vi "App - analyze RUS V6.vi"() -> ()   [LabVIEW 2021]
uses:
  lorentzian.ctl
  temperature sweep point.ctl
  <vilib>/Utility/miscctls.llb/LVCursorListTypeDef.ctl
  circle corners.ctl
  cursor window action.ctl
  find peak action.ctl
  follow the peak action.ctl
  slide action.ctl
  save-read action.ctl
  <vilib>/Utility/file.llb/Write To Spreadsheet File (string).vi
  complex region.ctl
  wavepacket.ctl
  cursor winow.ctl
  <vilib>/event_ctls.llb/eventvkey.ctl
  sweep file name.ctl
  single fit parameters.ctl
  omega map parameters.ctl
  plot scale state.ctl
  scale - offset gauge.ctl
  tfolder -- monotonic segment.ctl
  tfolder.ctl
  <vilib>/event_ctls.llb/lveventtype.ctl
  filter method control.ctl
  fit function selector control.ctl
  plot refs -- filter related.ctl
  peak -- parameters -- complex fit.ctl
  follow the peak control.ctl
  old slider control.ctl
  freq file read-write control.ctl
  read scan file control.ctl
panel:
  in  "magn field(T)":dbl format="%#.5f"
  in  "time (min)":dbl=1009.2833333313465
  in  "temperature(K)":dbl=69.845 format="%#.5f"
  in  "Tab : slide parameters":T1(tab)=enum."temperature folder related"
  in  "read scan file options":T2={"# columns"=3, "create bin file"=TRUE, "do not filter"=TRUE, "normalize phase"=TRUE, "read freq units"=enum."kHz"}
  in  "mapping: All":T3(ring)
  in  "slide control":T4={"in slide"=FALSE, "direction"=TRUE, "start "=FALSE, "stop"=FALSE, "next"=FALSE}
  in  "fit using":T5=enum."hyperbola"
  in  "mapping freq/gamma vs T":T3(ring)
  in  "mapping delta f vs T":T3(ring)
  in  "save/read":T6={"write to a file list"=0, "from file "="664_a", "erase"=FALSE, "load"=TRUE, "save"=TRUE, "to a file "="664_a", "read from file list"=0} {"read from file list" items=["664_a", "956_a", "1090_a"]}
  in  "follow the peak":T7={"factor"=20.0, "omega ?"=TRUE, "gamma ?"=FALSE, "max (kHz)"=30.0, "is clean"=FALSE, "acceptance"=0.5, "history - length"=10}
  in  "Tab : everything":T8(tab)
  in  "Tab : temperature folder":T9(tab)
  in  "plot when in slide":bool=TRUE
  in  "scale gauge: frequency vs T":dbl(slide)=0.9193548387096774 min=0.0 max=1.0 step=0.01 scale=0.0..1.0 scale format="%#_2g"
  out "Plot: frequency vs T":cluster{dbl[], dbl[]}[](graph)=[{array[1661 elements], array[1661 elements]}, {[14.503, 14.496, 14.494, 14.494, 14.485, 14.485, 14.487, 14.486, 14.479, 14.477, 14.476, 14.474, 14.473, 14.478, 14.475, 14.47, 14.472, 14.471, 14.469, 14.466, 14.467, 14.468, 14.463, 14.464, 14.462, 14.457, 14.457, 14.456, 14.45, 14.449, 14.446, 14.451, 14.451, 14.448, 14.449, 14.451, 14.449, 14.445, 14.447, 14.443, 14.439, 14.439, 14.439, 14.439, 14.44, 14.433, 14.434, 14.43, 14.43, 14.43, 14.434, 14.434, 14.431, 14.429, 14.426, 14.429, 14.429, 14.425, 14.426, 14.422, 14.424, 14.421, 14.418, 14.417, 14.415, 14.413, 14.414, 14.412, 14.418, 14.417, 14.412, 14.413, 14.41, 14.414, 14.408, 14.407, 14.406, 14.402, 14.4, 14.396, 14.394, 14.393, 14.39, 14.387, 14.39, 14.385, 14.384, 14.387, 14.388, 14.382, 14.384, 14.381, 14.381, 14.376, 14.375, 14.371, 14.371, 14.369, 14.369, 14.373, 14.37, 14.368, 14.366, 14.363, 14.364, 14.367, 14.363, 14.363, 14.363, 14.36, 14.361, 14.361, 14.357, 14.357, 14.355, 14.354, 14.354, 14.352, 14.349, 14.353, 14.35, 14.351, 14.351, 14.353, 14.352, 14.354, 14.354, 14.358, 14.357, 14.356, 14.356, 14.354, 14.35, 14.352, 14.354, 14.349, 14.349, 14.346], [0.0, 0.0, 0.0, 0.0, 0.0, 0.0, 0.0, 0.0, 0.0, 0.0, 0.0, 0.0, 0.0, 0.0, 0.0, 0.0, 0.0, 0.0, 0.0, 0.0, 0.0, 0.0, 0.0, 0.0, 0.0, 0.0, 0.0, 0.0, 0.0, 0.0, 0.0, 0.0, 0.0, 0.0, 0.0, 0.0, 0.0, 0.0, 0.0, 0.0, 0.0, 0.0, 0.0, 0.0, 0.0, 0.0, 0.0, 0.0, 0.0, 0.0, 0.0, 0.0, 0.0, 0.0, 0.0, 0.0, 0.0, 0.0, 0.0, 0.0, 0.0, 0.0, 0.0, 0.0, 0.0, 0.0, 0.0, 0.0, 0.0, 0.0, 0.0, 0.0, 0.0, 0.0, 0.0, 0.0, 0.0, 0.0, 0.0, 0.0, 0.0, 0.0, 0.0, 0.0, 0.0, 0.0, 0.0, 0.0, 0.0, 0.0, 0.0, 0.0, 0.0, 0.0, 0.0, 0.0, 0.0, 0.0, 0.0, 0.0, 0.0, 0.0, 0.0, 0.0, 0.0, 0.0, 0.0, 0.0, 0.0, 0.0, 0.0, 0.0, 0.0, 0.0, 0.0, 0.0, 0.0, 0.0, 0.0, 0.0, 0.0, 0.0, 0.0, 0.0, 0.0, 0.0, 0.0, 0.0, 0.0, 0.0, 0.0, 0.0, 0.0, 0.0, 0.0, 0.0, 0.0, 0.0]}, {[14.344, 14.346, 14.346, 14.348, 14.353, 14.355, 14.349, 14.351, 14.35, 14.347, 14.35, 14.349, 14.35, 14.351, 14.351, 14.352, 14.351, 14.35, 14.353, 14.354, 14.356, 14.359, 14.361, 14.36, 14.364, 14.363, 14.368, 14.367, 14.368, 14.368, 14.366, 14.369, 14.369, 14.371, 14.377, 14.377, 14.374, 14.374, 14.376, 14.375, 14.379, 14.38, 14.384, 14.382, 14.383, 14.382, 14.381, 14.386, 14.389, 14.392, 14.395, 14.397, 14.399, 14.4, 14.404, 14.405, 14.407, 14.411, 14.416, 14.42, 14.42, 14.42, 14.42, 14.426, 14.427, 14.431, 14.43, 14.431, 14.433, 14.438, 14.434, 14.438, 14.441, 14.441, 14.444, 14.44, 14.446, 14.449, 14.447, 14.448, 14.453, 14.45, 14.451, 14.449, 14.45, 14.453, 14.455, 14.456, 14.457, 14.458, 14.455, 14.459, 14.46, 14.459, 14.461, 14.465, 14.467, 14.467, 14.469, 14.467, 14.467, 14.469, 14.471, 14.473, 14.47, 14.474, 14.471, 14.471, 14.473, 14.476, 14.477, 14.479, 14.481, 14.481, 14.483, 14.483, 14.484, 14.488, 14.49, 14.491, 14.493, 14.491, 14.489, 14.491, 14.492, 14.492, 14.496, 14.498, 14.495, 14.498, 14.496, 14.503, 14.504, 14.507, 14.507, 14.508, 14.507, 14.507, 14.508, 14.509, 14.511, 14.513, 14.511, 14.512, 14.512, 14.51, 14.511, 14.511, 14.511, 14.512, 14.517, 14.515, 14.518, 14.517, 14.517, 14.518, 14.518, 14.52, 14.525, 14.521, 14.524, 14.524, 14.524, 14.523, 14.527, 14.522, 14.52, 14.522, 14.526, 14.529, 14.531, 14.534, 14.533, 14.534, 14.532, 14.536, 14.538, 14.541, 14.544, 14.545, 14.542, 14.546, 14.547, 14.544, 14.549, 14.546, 14.55, 14.556, 14.554, 14.553, 14.556, 14.556, 14.56, 14.56, 14.561, 14.562, 14.56, 14.56, 14.561, 14.563, 14.564, 14.572, 14.568, 14.565, 14.569, 14.577, 14.571, 14.58, 14.578, 14.579, 14.581, 14.58, 14.577, 14.58, 14.583, 14.582, 14.584, 14.584, 14.585, 14.585, 14.585, 14.585, 14.587, 14.593, 14.595, 14.597, 14.595, 14.597, 14.595, 14.597, 14.597, 14.599, 14.599, 14.599, 14.601, 14.605, 14.604, 14.606, 14.606, 14.609, 14.613, 14.614, 14.619, 14.618, 14.62, 14.621, 14.623, 14.624, 14.628, 14.625, 14.628, 14.63, 14.63, 14.635, 14.636, 14.637, 14.639, 14.64, 14.641, 14.644, 14.65, 14.65, 14.654, 14.654, 14.657, 14.659, 14.66, 14.661, 14.664, 14.668, 14.669, 14.673, 14.673, 14.673, 14.676, 14.678, 14.678, 14.681, 14.682, 14.685, 14.689, 14.687, 14.688, 14.693, 14.693, 14.696, 14.697, 14.697, 14.699, 14.702, 14.706, 14.708, 14.703, 14.705, 14.708, 14.709, 14.714, 14.719, 14.717, 14.723, 14.725, 14.727, 14.732, 14.737, 14.737, 14.739, 14.744, 14.747, 14.75, 14.751, 14.757, 14.754, 14.762, 14.757, 14.761, 14.768, 14.764, 14.769, 14.773, 14.772, 14.778, 14.778, 14.778, 14.784, 14.784, 14.784, 14.789, 14.788, 14.791, 14.793, 14.796, 14.797, 14.8, 14.807, 14.806, 14.808, 14.812, 14.814, 14.82, 14.816], [0.0, 0.0, 0.0, 0.0, 0.0, 0.0, 0.0, 0.0, 0.0, 0.0, 0.0, 0.0, 0.0, 0.0, 0.0, 0.0, 0.0, 0.0, 0.0, 0.0, 0.0, 0.0, 0.0, 0.0, 0.0, 0.0, 0.0, 0.0, 0.0, 0.0, 0.0, 0.0, 0.0, 0.0, 0.0, 0.0, 0.0, 0.0, 0.0, 0.0, 0.0, 0.0, 0.0, 0.0, 0.0, 0.0, 0.0, 0.0, 0.0, 0.0, 0.0, 0.0, 0.0, 0.0, 0.0, 0.0, 0.0, 0.0, 0.0, 0.0, 0.0, 0.0, 0.0, 0.0, 0.0, 0.0, 0.0, 0.0, 0.0, 0.0, 0.0, 0.0, 0.0, 0.0, 0.0, 0.0, 0.0, 0.0, 0.0, 0.0, 0.0, 0.0, 0.0, 0.0, 0.0, 0.0, 0.0, 0.0, 0.0, 0.0, 0.0, 0.0, 0.0, 0.0, 0.0, 0.0, 0.0, 0.0, 0.0, 0.0, 0.0, 0.0, 0.0, 0.0, 0.0, 0.0, 0.0, 0.0, 0.0, 0.0, 0.0, 0.0, 0.0, 0.0, 0.0, 0.0, 0.0, 0.0, 0.0, 0.0, 0.0, 0.0, 0.0, 0.0, 0.0, 0.0, 0.0, 0.0, 0.0, 0.0, 0.0, 0.0, 0.0, 0.0, 0.0, 0.0, 0.0, 0.0, 0.0, 0.0, 0.0, 0.0, 0.0, 0.0, 0.0, 0.0, 0.0, 0.0, 0.0, 0.0, 0.0, 0.0, 0.0, 0.0, 0.0, 0.0, 0.0, 0.0, 0.0, 0.0, 0.0, 0.0, 0.0, 0.0, 0.0, 0.0, 0.0, 0.0, 0.0, 0.0, 0.0, 0.0, 0.0, 0.0, 0.0, 0.0, 0.0, 0.0, 0.0, 0.0, 0.0, 0.0, 0.0, 0.0, 0.0, 0.0, 0.0, 0.0, 0.0, 0.0, 0.0, 0.0, 0.0, 0.0, 0.0, 0.0, 0.0, 0.0, 0.0, 0.0, 0.0, 0.0, 0.0, 0.0, 0.0, 0.0, 0.0, 0.0, 0.0, 0.0, 0.0, 0.0, 0.0, 0.0, 0.0, 0.0, 0.0, 0.0, 0.0, 0.0, 0.0, 0.0, 0.0, 0.0, 0.0, 0.0, 0.0, 0.0, 0.0, 0.0, 0.0, 0.0, 0.0, 0.0, 0.0, 0.0, 0.0, 0.0, 0.0, 0.0, 0.0, 0.0, 0.0, 0.0, 0.0, 0.0, 0.0, 0.0, 0.0, 0.0, 0.0, 0.0, 0.0, 0.0, 0.0, 0.0, 0.0, 0.0, 0.0, 0.0, 0.0, 0.0, 0.0, 0.0, 0.0, 0.0, 0.0, 0.0, 0.0, 0.0, 0.0, 0.0, 0.0, 0.0, 0.0, 0.0, 0.0, 0.0, 0.0, 0.0, 0.0, 0.0, 0.0, 0.0, 0.0, 0.0, 0.0, 0.0, 0.0, 0.0, 0.0, 0.0, 0.0, 0.0, 0.0, 0.0, 0.0, 0.0, 0.0, 0.0, 0.0, 0.0, 0.0, 0.0, 0.0, 0.0, 0.0, 0.0, 0.0, 0.0, 0.0, 0.0, 0.0, 0.0, 0.0, 0.0, 0.0, 0.0, 0.0, 0.0, 0.0, 0.0, 0.0, 0.0, 0.0, 0.0, 0.0, 0.0, 0.0, 0.0, 0.0, 0.0, 0.0, 0.0, 0.0, 0.0, 0.0, 0.0, 0.0, 0.0]}]
  out "Plot: attenuation vs T":cluster{dbl[], dbl[]}[](graph)=[{array[1661 elements], array[1661 elements]}, {[14.503, 14.496, 14.494, 14.494, 14.485, 14.485, 14.487, 14.486, 14.479, 14.477, 14.476, 14.474, 14.473, 14.478, 14.475, 14.47, 14.472, 14.471, 14.469, 14.466, 14.467, 14.468, 14.463, 14.464, 14.462, 14.457, 14.457, 14.456, 14.45, 14.449, 14.446, 14.451, 14.451, 14.448, 14.449, 14.451, 14.449, 14.445, 14.447, 14.443, 14.439, 14.439, 14.439, 14.439, 14.44, 14.433, 14.434, 14.43, 14.43, 14.43, 14.434, 14.434, 14.431, 14.429, 14.426, 14.429, 14.429, 14.425, 14.426, 14.422, 14.424, 14.421, 14.418, 14.417, 14.415, 14.413, 14.414, 14.412, 14.418, 14.417, 14.412, 14.413, 14.41, 14.414, 14.408, 14.407, 14.406, 14.402, 14.4, 14.396, 14.394, 14.393, 14.39, 14.387, 14.39, 14.385, 14.384, 14.387, 14.388, 14.382, 14.384, 14.381, 14.381, 14.376, 14.375, 14.371, 14.371, 14.369, 14.369, 14.373, 14.37, 14.368, 14.366, 14.363, 14.364, 14.367, 14.363, 14.363, 14.363, 14.36, 14.361, 14.361, 14.357, 14.357, 14.355, 14.354, 14.354, 14.352, 14.349, 14.353, 14.35, 14.351, 14.351, 14.353, 14.352, 14.354, 14.354, 14.358, 14.357, 14.356, 14.356, 14.354, 14.35, 14.352, 14.354, 14.349, 14.349, 14.346], [0.0, 0.0, 0.0, 0.0, 0.0, 0.0, 0.0, 0.0, 0.0, 0.0, 0.0, 0.0, 0.0, 0.0, 0.0, 0.0, 0.0, 0.0, 0.0, 0.0, 0.0, 0.0, 0.0, 0.0, 0.0, 0.0, 0.0, 0.0, 0.0, 0.0, 0.0, 0.0, 0.0, 0.0, 0.0, 0.0, 0.0, 0.0, 0.0, 0.0, 0.0, 0.0, 0.0, 0.0, 0.0, 0.0, 0.0, 0.0, 0.0, 0.0, 0.0, 0.0, 0.0, 0.0, 0.0, 0.0, 0.0, 0.0, 0.0, 0.0, 0.0, 0.0, 0.0, 0.0, 0.0, 0.0, 0.0, 0.0, 0.0, 0.0, 0.0, 0.0, 0.0, 0.0, 0.0, 0.0, 0.0, 0.0, 0.0, 0.0, 0.0, 0.0, 0.0, 0.0, 0.0, 0.0, 0.0, 0.0, 0.0, 0.0, 0.0, 0.0, 0.0, 0.0, 0.0, 0.0, 0.0, 0.0, 0.0, 0.0, 0.0, 0.0, 0.0, 0.0, 0.0, 0.0, 0.0, 0.0, 0.0, 0.0, 0.0, 0.0, 0.0, 0.0, 0.0, 0.0, 0.0, 0.0, 0.0, 0.0, 0.0, 0.0, 0.0, 0.0, 0.0, 0.0, 0.0, 0.0, 0.0, 0.0, 0.0, 0.0, 0.0, 0.0, 0.0, 0.0, 0.0, 0.0]}, {[14.344, 14.346, 14.346, 14.348, 14.353, 14.355, 14.349, 14.351, 14.35, 14.347, 14.35, 14.349, 14.35, 14.351, 14.351, 14.352, 14.351, 14.35, 14.353, 14.354, 14.356, 14.359, 14.361, 14.36, 14.364, 14.363, 14.368, 14.367, 14.368, 14.368, 14.366, 14.369, 14.369, 14.371, 14.377, 14.377, 14.374, 14.374, 14.376, 14.375, 14.379, 14.38, 14.384, 14.382, 14.383, 14.382, 14.381, 14.386, 14.389, 14.392, 14.395, 14.397, 14.399, 14.4, 14.404, 14.405, 14.407, 14.411, 14.416, 14.42, 14.42, 14.42, 14.42, 14.426, 14.427, 14.431, 14.43, 14.431, 14.433, 14.438, 14.434, 14.438, 14.441, 14.441, 14.444, 14.44, 14.446, 14.449, 14.447, 14.448, 14.453, 14.45, 14.451, 14.449, 14.45, 14.453, 14.455, 14.456, 14.457, 14.458, 14.455, 14.459, 14.46, 14.459, 14.461, 14.465, 14.467, 14.467, 14.469, 14.467, 14.467, 14.469, 14.471, 14.473, 14.47, 14.474, 14.471, 14.471, 14.473, 14.476, 14.477, 14.479, 14.481, 14.481, 14.483, 14.483, 14.484, 14.488, 14.49, 14.491, 14.493, 14.491, 14.489, 14.491, 14.492, 14.492, 14.496, 14.498, 14.495, 14.498, 14.496, 14.503, 14.504, 14.507, 14.507, 14.508, 14.507, 14.507, 14.508, 14.509, 14.511, 14.513, 14.511, 14.512, 14.512, 14.51, 14.511, 14.511, 14.511, 14.512, 14.517, 14.515, 14.518, 14.517, 14.517, 14.518, 14.518, 14.52, 14.525, 14.521, 14.524, 14.524, 14.524, 14.523, 14.527, 14.522, 14.52, 14.522, 14.526, 14.529, 14.531, 14.534, 14.533, 14.534, 14.532, 14.536, 14.538, 14.541, 14.544, 14.545, 14.542, 14.546, 14.547, 14.544, 14.549, 14.546, 14.55, 14.556, 14.554, 14.553, 14.556, 14.556, 14.56, 14.56, 14.561, 14.562, 14.56, 14.56, 14.561, 14.563, 14.564, 14.572, 14.568, 14.565, 14.569, 14.577, 14.571, 14.58, 14.578, 14.579, 14.581, 14.58, 14.577, 14.58, 14.583, 14.582, 14.584, 14.584, 14.585, 14.585, 14.585, 14.585, 14.587, 14.593, 14.595, 14.597, 14.595, 14.597, 14.595, 14.597, 14.597, 14.599, 14.599, 14.599, 14.601, 14.605, 14.604, 14.606, 14.606, 14.609, 14.613, 14.614, 14.619, 14.618, 14.62, 14.621, 14.623, 14.624, 14.628, 14.625, 14.628, 14.63, 14.63, 14.635, 14.636, 14.637, 14.639, 14.64, 14.641, 14.644, 14.65, 14.65, 14.654, 14.654, 14.657, 14.659, 14.66, 14.661, 14.664, 14.668, 14.669, 14.673, 14.673, 14.673, 14.676, 14.678, 14.678, 14.681, 14.682, 14.685, 14.689, 14.687, 14.688, 14.693, 14.693, 14.696, 14.697, 14.697, 14.699, 14.702, 14.706, 14.708, 14.703, 14.705, 14.708, 14.709, 14.714, 14.719, 14.717, 14.723, 14.725, 14.727, 14.732, 14.737, 14.737, 14.739, 14.744, 14.747, 14.75, 14.751, 14.757, 14.754, 14.762, 14.757, 14.761, 14.768, 14.764, 14.769, 14.773, 14.772, 14.778, 14.778, 14.778, 14.784, 14.784, 14.784, 14.789, 14.788, 14.791, 14.793, 14.796, 14.797, 14.8, 14.807, 14.806, 14.808, 14.812, 14.814, 14.82, 14.816], [0.0, 0.0, 0.0, 0.0, 0.0, 0.0, 0.0, 0.0, 0.0, 0.0, 0.0, 0.0, 0.0, 0.0, 0.0, 0.0, 0.0, 0.0, 0.0, 0.0, 0.0, 0.0, 0.0, 0.0, 0.0, 0.0, 0.0, 0.0, 0.0, 0.0, 0.0, 0.0, 0.0, 0.0, 0.0, 0.0, 0.0, 0.0, 0.0, 0.0, 0.0, 0.0, 0.0, 0.0, 0.0, 0.0, 0.0, 0.0, 0.0, 0.0, 0.0, 0.0, 0.0, 0.0, 0.0, 0.0, 0.0, 0.0, 0.0, 0.0, 0.0, 0.0, 0.0, 0.0, 0.0, 0.0, 0.0, 0.0, 0.0, 0.0, 0.0, 0.0, 0.0, 0.0, 0.0, 0.0, 0.0, 0.0, 0.0, 0.0, 0.0, 0.0, 0.0, 0.0, 0.0, 0.0, 0.0, 0.0, 0.0, 0.0, 0.0, 0.0, 0.0, 0.0, 0.0, 0.0, 0.0, 0.0, 0.0, 0.0, 0.0, 0.0, 0.0, 0.0, 0.0, 0.0, 0.0, 0.0, 0.0, 0.0, 0.0, 0.0, 0.0, 0.0, 0.0, 0.0, 0.0, 0.0, 0.0, 0.0, 0.0, 0.0, 0.0, 0.0, 0.0, 0.0, 0.0, 0.0, 0.0, 0.0, 0.0, 0.0, 0.0, 0.0, 0.0, 0.0, 0.0, 0.0, 0.0, 0.0, 0.0, 0.0, 0.0, 0.0, 0.0, 0.0, 0.0, 0.0, 0.0, 0.0, 0.0, 0.0, 0.0, 0.0, 0.0, 0.0, 0.0, 0.0, 0.0, 0.0, 0.0, 0.0, 0.0, 0.0, 0.0, 0.0, 0.0, 0.0, 0.0, 0.0, 0.0, 0.0, 0.0, 0.0, 0.0, 0.0, 0.0, 0.0, 0.0, 0.0, 0.0, 0.0, 0.0, 0.0, 0.0, 0.0, 0.0, 0.0, 0.0, 0.0, 0.0, 0.0, 0.0, 0.0, 0.0, 0.0, 0.0, 0.0, 0.0, 0.0, 0.0, 0.0, 0.0, 0.0, 0.0, 0.0, 0.0, 0.0, 0.0, 0.0, 0.0, 0.0, 0.0, 0.0, 0.0, 0.0, 0.0, 0.0, 0.0, 0.0, 0.0, 0.0, 0.0, 0.0, 0.0, 0.0, 0.0, 0.0, 0.0, 0.0, 0.0, 0.0, 0.0, 0.0, 0.0, 0.0, 0.0, 0.0, 0.0, 0.0, 0.0, 0.0, 0.0, 0.0, 0.0, 0.0, 0.0, 0.0, 0.0, 0.0, 0.0, 0.0, 0.0, 0.0, 0.0, 0.0, 0.0, 0.0, 0.0, 0.0, 0.0, 0.0, 0.0, 0.0, 0.0, 0.0, 0.0, 0.0, 0.0, 0.0, 0.0, 0.0, 0.0, 0.0, 0.0, 0.0, 0.0, 0.0, 0.0, 0.0, 0.0, 0.0, 0.0, 0.0, 0.0, 0.0, 0.0, 0.0, 0.0, 0.0, 0.0, 0.0, 0.0, 0.0, 0.0, 0.0, 0.0, 0.0, 0.0, 0.0, 0.0, 0.0, 0.0, 0.0, 0.0, 0.0, 0.0, 0.0, 0.0, 0.0, 0.0, 0.0, 0.0, 0.0, 0.0, 0.0, 0.0, 0.0, 0.0, 0.0, 0.0, 0.0, 0.0, 0.0, 0.0, 0.0, 0.0, 0.0, 0.0, 0.0, 0.0, 0.0, 0.0, 0.0, 0.0, 0.0, 0.0, 0.0, 0.0, 0.0]}]
  in  "Sweep folder path":path=path "D:/Data/Ultrasound/LSCO/LSCO22__130814c/5_Cooling_2nd_try"
  out "Plot: Time":cluster{dbl[], dbl[]}[](graph)
  out "Plot: delta f":cluster{dbl[], dbl[]}[](graph)=[{array[1661 elements], array[1661 elements]}, {[14.503, 14.496, 14.494, 14.494, 14.485, 14.485, 14.487, 14.486, 14.479, 14.477, 14.476, 14.474, 14.473, 14.478, 14.475, 14.47, 14.472, 14.471, 14.469, 14.466, 14.467, 14.468, 14.463, 14.464, 14.462, 14.457, 14.457, 14.456, 14.45, 14.449, 14.446, 14.451, 14.451, 14.448, 14.449, 14.451, 14.449, 14.445, 14.447, 14.443, 14.439, 14.439, 14.439, 14.439, 14.44, 14.433, 14.434, 14.43, 14.43, 14.43, 14.434, 14.434, 14.431, 14.429, 14.426, 14.429, 14.429, 14.425, 14.426, 14.422, 14.424, 14.421, 14.418, 14.417, 14.415, 14.413, 14.414, 14.412, 14.418, 14.417, 14.412, 14.413, 14.41, 14.414, 14.408, 14.407, 14.406, 14.402, 14.4, 14.396, 14.394, 14.393, 14.39, 14.387, 14.39, 14.385, 14.384, 14.387, 14.388, 14.382, 14.384, 14.381, 14.381, 14.376, 14.375, 14.371, 14.371, 14.369, 14.369, 14.373, 14.37, 14.368, 14.366, 14.363, 14.364, 14.367, 14.363, 14.363, 14.363, 14.36, 14.361, 14.361, 14.357, 14.357, 14.355, 14.354, 14.354, 14.352, 14.349, 14.353, 14.35, 14.351, 14.351, 14.353, 14.352, 14.354, 14.354, 14.358, 14.357, 14.356, 14.356, 14.354, 14.35, 14.352, 14.354, 14.349, 14.349, 14.346], [nan, nan, nan, nan, nan, nan, nan, nan, nan, nan, nan, nan, nan, nan, nan, nan, nan, nan, nan, nan, nan, nan, nan, nan, nan, nan, nan, nan, nan, nan, nan, nan, nan, nan, nan, nan, nan, nan, nan, nan, nan, nan, nan, nan, nan, nan, nan, nan, nan, nan, nan, nan, nan, nan, nan, nan, nan, nan, nan, nan, nan, nan, nan, nan, nan, nan, nan, nan, nan, nan, nan, nan, nan, nan, nan, nan, nan, nan, nan, nan, nan, nan, nan, nan, nan, nan, nan, nan, nan, nan, nan, nan, nan, nan, nan, nan, nan, nan, nan, nan, nan, nan, nan, nan, nan, nan, nan, nan, nan, nan, nan, nan, nan, nan, nan, nan, nan, nan, nan, nan, nan, nan, nan, nan, nan, nan, nan, nan, nan, nan, nan, nan, nan, nan, nan, nan, nan, nan]}, {[14.344, 14.346, 14.346, 14.348, 14.353, 14.355, 14.349, 14.351, 14.35, 14.347, 14.35, 14.349, 14.35, 14.351, 14.351, 14.352, 14.351, 14.35, 14.353, 14.354, 14.356, 14.359, 14.361, 14.36, 14.364, 14.363, 14.368, 14.367, 14.368, 14.368, 14.366, 14.369, 14.369, 14.371, 14.377, 14.377, 14.374, 14.374, 14.376, 14.375, 14.379, 14.38, 14.384, 14.382, 14.383, 14.382, 14.381, 14.386, 14.389, 14.392, 14.395, 14.397, 14.399, 14.4, 14.404, 14.405, 14.407, 14.411, 14.416, 14.42, 14.42, 14.42, 14.42, 14.426, 14.427, 14.431, 14.43, 14.431, 14.433, 14.438, 14.434, 14.438, 14.441, 14.441, 14.444, 14.44, 14.446, 14.449, 14.447, 14.448, 14.453, 14.45, 14.451, 14.449, 14.45, 14.453, 14.455, 14.456, 14.457, 14.458, 14.455, 14.459, 14.46, 14.459, 14.461, 14.465, 14.467, 14.467, 14.469, 14.467, 14.467, 14.469, 14.471, 14.473, 14.47, 14.474, 14.471, 14.471, 14.473, 14.476, 14.477, 14.479, 14.481, 14.481, 14.483, 14.483, 14.484, 14.488, 14.49, 14.491, 14.493, 14.491, 14.489, 14.491, 14.492, 14.492, 14.496, 14.498, 14.495, 14.498, 14.496, 14.503, 14.504, 14.507, 14.507, 14.508, 14.507, 14.507, 14.508, 14.509, 14.511, 14.513, 14.511, 14.512, 14.512, 14.51, 14.511, 14.511, 14.511, 14.512, 14.517, 14.515, 14.518, 14.517, 14.517, 14.518, 14.518, 14.52, 14.525, 14.521, 14.524, 14.524, 14.524, 14.523, 14.527, 14.522, 14.52, 14.522, 14.526, 14.529, 14.531, 14.534, 14.533, 14.534, 14.532, 14.536, 14.538, 14.541, 14.544, 14.545, 14.542, 14.546, 14.547, 14.544, 14.549, 14.546, 14.55, 14.556, 14.554, 14.553, 14.556, 14.556, 14.56, 14.56, 14.561, 14.562, 14.56, 14.56, 14.561, 14.563, 14.564, 14.572, 14.568, 14.565, 14.569, 14.577, 14.571, 14.58, 14.578, 14.579, 14.581, 14.58, 14.577, 14.58, 14.583, 14.582, 14.584, 14.584, 14.585, 14.585, 14.585, 14.585, 14.587, 14.593, 14.595, 14.597, 14.595, 14.597, 14.595, 14.597, 14.597, 14.599, 14.599, 14.599, 14.601, 14.605, 14.604, 14.606, 14.606, 14.609, 14.613, 14.614, 14.619, 14.618, 14.62, 14.621, 14.623, 14.624, 14.628, 14.625, 14.628, 14.63, 14.63, 14.635, 14.636, 14.637, 14.639, 14.64, 14.641, 14.644, 14.65, 14.65, 14.654, 14.654, 14.657, 14.659, 14.66, 14.661, 14.664, 14.668, 14.669, 14.673, 14.673, 14.673, 14.676, 14.678, 14.678, 14.681, 14.682, 14.685, 14.689, 14.687, 14.688, 14.693, 14.693, 14.696, 14.697, 14.697, 14.699, 14.702, 14.706, 14.708, 14.703, 14.705, 14.708, 14.709, 14.714, 14.719, 14.717, 14.723, 14.725, 14.727, 14.732, 14.737, 14.737, 14.739, 14.744, 14.747, 14.75, 14.751, 14.757, 14.754, 14.762, 14.757, 14.761, 14.768, 14.764, 14.769, 14.773, 14.772, 14.778, 14.778, 14.778, 14.784, 14.784, 14.784, 14.789, 14.788, 14.791, 14.793, 14.796, 14.797, 14.8, 14.807, 14.806, 14.808, 14.812, 14.814, 14.82, 14.816], [nan, nan, nan, nan, nan, nan, nan, nan, nan, nan, nan, nan, nan, nan, nan, nan, nan, nan, nan, nan, nan, nan, nan, nan, nan, nan, nan, nan, nan, nan, nan, nan, nan, nan, nan, nan, nan, nan, nan, nan, nan, nan, nan, nan, nan, nan, nan, nan, nan, nan, nan, nan, nan, nan, nan, nan, nan, nan, nan, nan, nan, nan, nan, nan, nan, nan, nan, nan, nan, nan, nan, nan, nan, nan, nan, nan, nan, nan, nan, nan, nan, nan, nan, nan, nan, nan, nan, nan, nan, nan, nan, nan, nan, nan, nan, nan, nan, nan, nan, nan, nan, nan, nan, nan, nan, nan, nan, nan, nan, nan, nan, nan, nan, nan, nan, nan, nan, nan, nan, nan, nan, nan, nan, nan, nan, nan, nan, nan, nan, nan, nan, nan, nan, nan, nan, nan, nan, nan, nan, nan, nan, nan, nan, nan, nan, nan, nan, nan, nan, nan, nan, nan, nan, nan, nan, nan, nan, nan, nan, nan, nan, nan, nan, nan, nan, nan, nan, nan, nan, nan, nan, nan, nan, nan, nan, nan, nan, nan, nan, nan, nan, nan, nan, nan, nan, nan, nan, nan, nan, nan, nan, nan, nan, nan, nan, nan, nan, nan, nan, nan, nan, nan, nan, nan, nan, nan, nan, nan, nan, nan, nan, nan, nan, nan, nan, nan, nan, nan, nan, nan, nan, nan, nan, nan, nan, nan, nan, nan, nan, nan, nan, nan, nan, nan, nan, nan, nan, nan, nan, nan, nan, nan, nan, nan, nan, nan, nan, nan, nan, nan, nan, nan, nan, nan, nan, nan, nan, nan, nan, nan, nan, nan, nan, nan, nan, nan, nan, nan, nan, nan, nan, nan, nan, nan, nan, nan, nan, nan, nan, nan, nan, nan, nan, nan, nan, nan, nan, nan, nan, nan, nan, nan, nan, nan, nan, nan, nan, nan, nan, nan, nan, nan, nan, nan, nan, nan, nan, nan, nan, nan, nan, nan, nan, nan, nan, nan, nan, nan, nan, nan, nan, nan, nan, nan, nan, nan, nan, nan, nan, nan, nan, nan, nan, nan, nan, nan, nan, nan, nan, nan]}]
  in  "scale gauge: delta f plot":dbl(slide)=0.4074074074074074 min=0.0 max=1.0 step=0.001 scale=0.001..1.0 scale format="%#_2f"
  in  "scale gauge: Attenuation vs T":T10={"scale offset"=1.0, "scale range"=1.0} {"scale range" min=0.0 max=1.0 step=1e-05 scale=0.001..1.0 scale format="%#_2g"; "scale offset" min=0.0 max=1.0 step=1e-05 scale=0.001..1.0 scale format="%#_2g"}
  in  "in sweep folder":bool=TRUE
  out "-- loading ...":bool=TRUE
  in  "monotonic segment":bool=TRUE
  out "section":i32=2
  in  "freq(T) : auto-adjust Y scale":bool=TRUE
  out "array of peaks":dbl[](array[numeric])
  out "Plot: JBBetts":cluster{"all rows":dbl[], "all rows":dbl[]}[](graph)
  in  "number of hits to threshold":i32=5
  in  "scan speed":i32=50
  in  "threshold window":dbl
  out "best fit parameters":dbl[](array[numeric])=[nan, nan, 100.0]
  in  "log-log":bool
  out "fit points after":i32
  in  "varshni win (relative)":dbl=1.25
  out "fit function name":string="fit function - hyperbola.vi"
  out "fit points before":i32
  out "Plot: df/dT":cluster{dbl[], dbl[]}[](graph)=[{[295.00000002, 295.00000003, 295.00000004, 295.00000005, 295.00000006, 295.00000007, 295.00000008, 295.00000009, 295.0000001, 295.00000011, 295.00000012, 295.00000013, 281.03000001, 280.53800001, 280.46900001, 280.39300001, 295.43400001, 295.74200001], [nan, nan, nan, nan, nan, nan, nan, nan, nan, nan, nan, nan, nan, nan, nan, nan, nan, nan]}, {array[506 elements], array[506 elements]}, {[9.93300002, 9.99610001, 10.52000001, 11.05600001, 11.61100001, 12.15100001, 12.69800001, 13.25100001, 13.80200001, 14.33000001, 14.86900001, 15.39200001, 15.93800001, 16.47000001, 17.00300001, 17.55000001, 18.07800001, 18.61000001, 19.13700001, 19.67900001], [-5.898501057178606, 0.40573480699278597, -0.01242680298650033, -0.014835847901034963, 0.0041007841953597055, 0.007500497934041738, -0.0036169475710465483, -0.004873529820569241, -0.001431716497795133, -0.0017305298150552936, 0.014952075312570624, 0.009745493927916953, 0.001853673862849577, -0.03608755144933456, 0.018359119142839025, -0.03278855296473742, 0.015014995288115491, 0.0102723685732519, 0.009671160088004945, -0.0005418936495686807]}]
  in  "scale gauge: df/dT plot":dbl(slide)=0.012345679012345678 min=0.0 max=10.0 step=0.01 scale=0.0..10.0 scale format="%#_2g"
  in  "zoom factor - derivative":i32=10
  in  "derivative window":i32=10
  in  "log T ?":bool
  out "Plot: attenuation vs H":cluster{dbl[], dbl[]}[](graph)
  out "Plot: frequency vs H":cluster{dbl[], dbl[]}[](graph)
  in  "scale gauge: frequency vs H":dbl(slide)=0.11290322580645161 min=0.0 max=1.0 step=0.01 scale=0.0..1.0 scale format="%#_2g"
  in  "scale gauge: Attenuation vs H":T10={"scale offset"=0.5005000000000001, "scale range"=0.07943} {"scale range" min=0.0 max=1.0 step=1e-05 scale=0.001..1.0 scale format="%#_2g"; "scale offset" min=0.0 max=1.0 step=1e-05 scale=0.001..1.0 scale format="%#_2g"}
  out "Plot: H vs Time":cluster{dbl[], dbl[]}[](graph)
  in  "Magn Field points":dbl[](array[numeric])
  in  "factor":dbl(slide) scale=0.5..50.0
  out "interpolated gamma":dbl=0.016725252746731926
  out "interpolated omega":dbl=662.9654599727345
  out "complex plane norm":dbl=0.007905574826145054
  out "complex plane center":cdb=0.027737603223116452+0.0034015268867928035i
  in  "fiter staff":bool
  out "Plot: frequency vs power":cluster{dbl[], dbl[]}[](graph)=[{array[1661 elements], array[1661 elements]}, {[2.1, 2.1, 2.1, 2.1, 2.1, 2.1, 2.1, 2.1, 2.1, 2.1, 2.1, 2.1, 2.1, 2.1, 2.1, 2.1, 2.1, 2.1, 2.1, 2.1, 2.1, 2.1, 2.1, 2.1, 2.1, 2.1, 2.1, 2.1, 2.1, 2.1, 2.1, 2.1, 2.1, 2.1, 2.1, 2.1, 2.1, 2.1, 2.1, 2.1, 2.1, 2.1, 2.1, 2.1, 2.1, 2.1, 2.1, 2.1, 2.1, 2.1, 2.1, 2.1, 2.1, 2.1, 2.1, 2.1, 2.1, 2.1, 2.1, 2.1, 2.1, 2.1, 2.1, 2.1, 2.1, 2.1, 2.1, 2.1, 2.1, 2.1, 2.1, 2.1, 2.1, 2.1, 2.1, 2.1, 2.1, 2.1, 2.1, 2.1, 2.1, 2.1, 2.1, 2.1, 2.1, 2.1, 2.1, 2.1, 2.1, 2.1, 2.1, 2.1, 2.1, 2.1, 2.1, 2.1, 2.1, 2.1, 2.1, 2.1, 2.1, 2.1, 2.1, 2.1, 2.1, 2.1, 2.1, 2.1, 2.1, 2.1, 2.1, 2.1, 2.1, 2.1, 2.1, 2.1, 2.1, 2.1, 2.1, 2.1, 2.1, 2.1, 2.1, 2.1, 2.1, 2.1, 2.1, 2.1, 2.1, 2.1, 2.1, 2.1, 2.1, 2.1, 2.1, 2.1, 2.1, 2.1], [0.0, 0.0, 0.0, 0.0, 0.0, 0.0, 0.0, 0.0, 0.0, 0.0, 0.0, 0.0, 0.0, 0.0, 0.0, 0.0, 0.0, 0.0, 0.0, 0.0, 0.0, 0.0, 0.0, 0.0, 0.0, 0.0, 0.0, 0.0, 0.0, 0.0, 0.0, 0.0, 0.0, 0.0, 0.0, 0.0, 0.0, 0.0, 0.0, 0.0, 0.0, 0.0, 0.0, 0.0, 0.0, 0.0, 0.0, 0.0, 0.0, 0.0, 0.0, 0.0, 0.0, 0.0, 0.0, 0.0, 0.0, 0.0, 0.0, 0.0, 0.0, 0.0, 0.0, 0.0, 0.0, 0.0, 0.0, 0.0, 0.0, 0.0, 0.0, 0.0, 0.0, 0.0, 0.0, 0.0, 0.0, 0.0, 0.0, 0.0, 0.0, 0.0, 0.0, 0.0, 0.0, 0.0, 0.0, 0.0, 0.0, 0.0, 0.0, 0.0, 0.0, 0.0, 0.0, 0.0, 0.0, 0.0, 0.0, 0.0, 0.0, 0.0, 0.0, 0.0, 0.0, 0.0, 0.0, 0.0, 0.0, 0.0, 0.0, 0.0, 0.0, 0.0, 0.0, 0.0, 0.0, 0.0, 0.0, 0.0, 0.0, 0.0, 0.0, 0.0, 0.0, 0.0, 0.0, 0.0, 0.0, 0.0, 0.0, 0.0, 0.0, 0.0, 0.0, 0.0, 0.0, 0.0]}, {[2.1, 2.1, 2.1, 2.1, 2.1, 2.1, 2.1, 2.1, 2.1, 2.1, 2.1, 2.1, 2.1, 2.1, 2.1, 2.1, 2.1, 2.1, 2.1, 2.1, 2.1, 2.1, 2.1, 2.1, 2.1, 2.1, 2.1, 2.1, 2.1, 2.1, 2.1, 2.1, 2.1, 2.1, 2.1, 2.1, 2.1, 2.1, 2.1, 2.1, 2.1, 2.1, 2.1, 2.1, 2.1, 2.1, 2.1, 2.1, 2.1, 2.1, 2.1, 2.1, 2.1, 2.1, 2.1, 2.1, 2.1, 2.1, 2.1, 2.1, 2.1, 2.1, 2.1, 2.1, 2.1, 2.1, 2.1, 2.1, 2.1, 2.1, 2.1, 2.1, 2.1, 2.1, 2.1, 2.1, 2.1, 2.1, 2.1, 2.1, 2.1, 2.1, 2.1, 2.1, 2.1, 2.1, 2.1, 2.1, 2.1, 2.1, 2.1, 2.1, 2.1, 2.1, 2.1, 2.1, 2.1, 2.1, 2.1, 2.1, 2.1, 2.1, 2.1, 2.1, 2.1, 2.1, 2.1, 2.1, 2.1, 2.1, 2.1, 2.1, 2.1, 2.1, 2.1, 2.1, 2.1, 2.1, 2.1, 2.1, 2.1, 2.1, 2.1, 2.1, 2.1, 2.1, 2.1, 2.1, 2.1, 2.1, 2.1, 2.1, 2.1, 2.1, 2.1, 2.1, 2.1, 2.1, 2.1, 2.1, 2.1, 2.1, 2.1, 2.1, 2.1, 2.1, 2.1, 2.1, 2.1, 2.1, 2.1, 2.1, 2.1, 2.1, 2.1, 2.1, 2.1, 2.1, 2.1, 2.1, 2.1, 2.1, 2.1, 2.1, 2.1, 2.1, 2.1, 2.1, 2.1, 2.1, 2.1, 2.1, 2.1, 2.1, 2.1, 2.1, 2.1, 2.1, 2.1, 2.1, 2.1, 2.1, 2.1, 2.1, 2.1, 2.1, 2.1, 2.1, 2.1, 2.1, 2.1, 2.1, 2.1, 2.1, 2.1, 2.1, 2.1, 2.1, 2.1, 2.1, 2.1, 2.1, 2.1, 2.1, 2.1, 2.1, 2.1, 2.1, 2.1, 2.1, 2.1, 2.1, 2.1, 2.1, 2.1, 2.1, 2.1, 2.1, 2.1, 2.1, 2.1, 2.1, 2.1, 2.1, 2.1, 2.1, 2.1, 2.1, 2.1, 2.1, 2.1, 2.1, 2.1, 2.1, 2.1, 2.1, 2.1, 2.1, 2.1, 2.1, 2.1, 2.1, 2.1, 2.1, 2.1, 2.1, 2.1, 2.1, 2.1, 2.1, 2.1, 2.1, 2.1, 2.1, 2.1, 2.1, 2.1, 2.1, 2.1, 2.1, 2.1, 2.1, 2.1, 2.1, 2.1, 2.1, 2.1, 2.1, 2.1, 2.1, 2.1, 2.1, 2.1, 2.1, 2.1, 2.1, 2.1, 2.1, 2.1, 2.1, 2.1, 2.1, 2.1, 2.1, 2.1, 2.1, 2.1, 2.1, 2.1, 2.1, 2.1, 2.1, 2.1, 2.1, 2.1, 2.1, 2.1, 2.1, 2.1, 2.1, 2.1, 2.1, 2.1, 2.1, 2.1, 2.1, 2.1, 2.1, 2.1, 2.1, 2.1, 2.1, 2.1, 2.1, 2.1, 2.1, 2.1, 2.1, 2.1, 2.1, 2.1, 2.1, 2.1, 2.1, 2.1, 2.1, 2.1, 2.1, 2.1, 2.1, 2.1, 2.1, 2.1, 2.1, 2.1, 2.1, 2.1, 2.1, 2.1, 2.1], [0.0, 0.0, 0.0, 0.0, 0.0, 0.0, 0.0, 0.0, 0.0, 0.0, 0.0, 0.0, 0.0, 0.0, 0.0, 0.0, 0.0, 0.0, 0.0, 0.0, 0.0, 0.0, 0.0, 0.0, 0.0, 0.0, 
